vi "821_M1.vi"() -> ()   [LabVIEW 2018]
panel:
  in  "启动开关":bool
  out "阀门2":bool
  in  "阀门1":bool
  in  "设定气压设定值":bool
  out "气压设定值":dbl=550.0
  out "M1气压数值":dbl(knob) scale=0.0..1000.0
  in  "进气流量":dbl(slide) scale=0.0..100.0
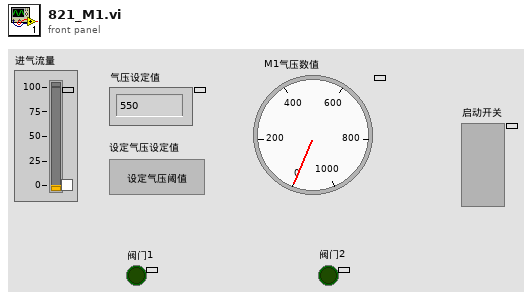
[diagram p1: front panel]
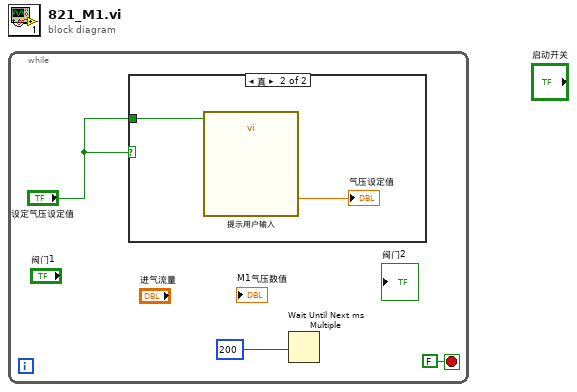
[diagram p0: block diagram]
diagram:
  n1 = while {
    stop <- FALSE stop-if-true
    n2 = case shown="真" "设定气压设定值" {
      tunnel: "设定气压设定值" -> [_ w4]
      frame False {
      }
      frame True {
        n3 = call "提示用户输入"("Enable"=w4) -> ("气压设定值"=→"气压设定值":dbl)  [unwired: 16 in, 2 out]
      }
    }
    n4 = Wait Until Next ms Multiple(millisecond multiple=200) -> ()  [unwired: 1 out]
  }
